vi "Default Settings.vi"(8 "error in (no error)":errorcluster, 11 "C4 Dispense in 2":refnum<class "6 Inch Iterative Dispense.lvclass">) -> (0 "error out":errorcluster, 3 "C4 Dispense out 2":refnum<class "6 Inch Iterative Dispense.lvclass">)   [LabVIEW 2016, in "6 Inch Iterative Dispense.lvclass"]
uses:
  6 Inch Iterative Dispense.lvclass
  D:/LabVIEW/20220413/UCSB-Gantry/V5/Classes/Routine/Dispense/Iterative Dispense/Iterative Dispense.lvclass
  D:/LabVIEW/20220413/UCSB-Gantry/V5/Classes/Routine/Dispense/Dispense.lvclass
  Iterative Dispense.lvclass/Iterative Dispense.ctl
  Read Speed.vi
  Read Number of Lines.vi
  Read Distance From Edges.vi
  Iterative Dispense.lvclass
  Dispense.lvclass
panel:
  # "This Routine does not Accept Settings"
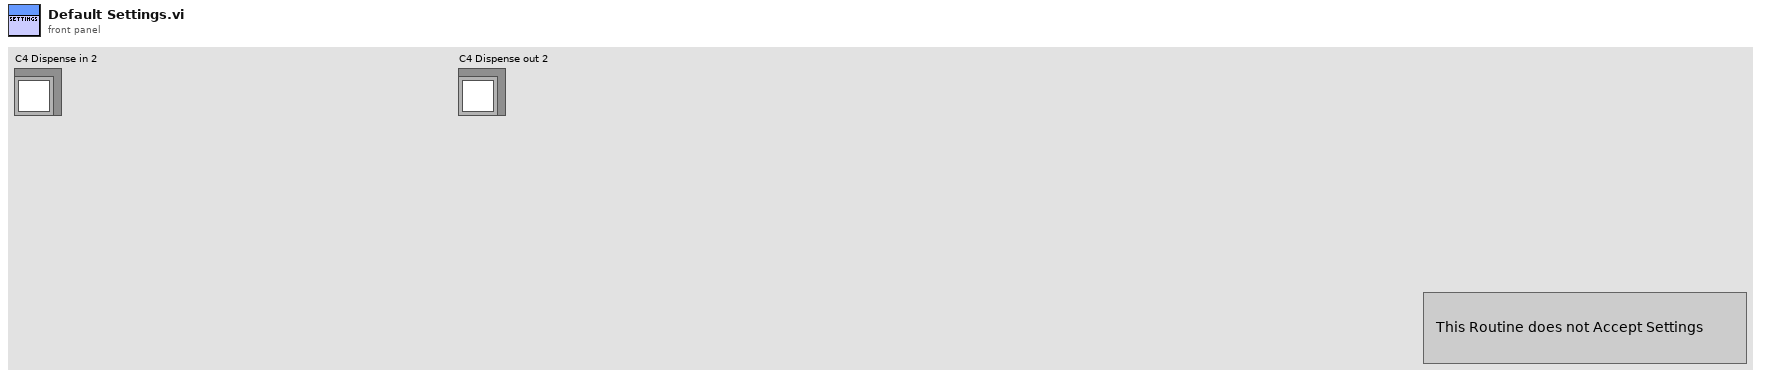
[diagram p1: front panel]
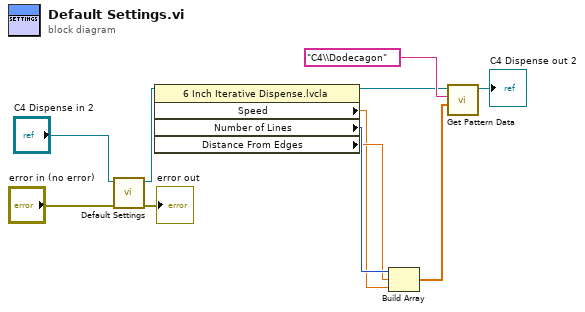
[diagram p0: block diagram]
diagram:
  n1 = call-parent "Default Settings.vi"("error in (no error)"="error in (no error)", "C4 Dispense in 2"="C4 Dispense in 2") -> ("error out"=→"error out":errorcluster, "C4 Dispense out 2"=w8:refnum<class "6 Inch Iterative Dispense.lvclass">)  [unwired: 8 in]
  n2 = property class="6 Inch Iterative Dispense.lvcla"(reference=w8) -> (reference out=w6:refnum<class "6 Inch Iterative Dispense.lvclass">, "Speed"=w2:dbl, "Number of Lines"=w4:i32, "Distance From Edges"=w3:dbl)  [unwired: 1 in, 1 out]
  n3 = Build Array(w4, w3, w2) -> (w1:dbl[])
  n4 = call "Get Pattern Data.vi"("File Name"=w1, "Folder Name"="C4\\Dodecagon", "Dispense.lvclass"=w6) -> ("Dispense Out"=→"C4 Dispense out 2":refnum<class "6 Inch Iterative Dispense.lvclass">)  [unwired: 8 in]
